vi "SW_Gen_2D_Histogram.vi"(7 "Picture reference in":refnum<vi>, 8 "Pixels per mm":dbl, 9 "Y coord array":dbl[](array[numeric]), 10 "X coord array":dbl[](array[numeric]), 11 "Bounds":T6) -> (1 "8-bit density map":u8[][](array[numeric]), 2 "24-bit pixmap":u32[][](array[numeric]), 3 "Picture":picture)   [LabVIEW 2018, in "Tracker.lvlib"]
uses:
  Tracker.lvlib
  <vilib>/Utility/miscctls.llb/LVBoundsTypeDef.ctl
  <vilib>/Heliosphere Research LLC/Advanced Plotting Toolkit/api_plotting/Histogram2DProperties.ctl
  <vilib>/Heliosphere Research LLC/Advanced Plotting Toolkit/properties/Colormap.ctl
  <vilib>/Heliosphere Research LLC/Advanced Plotting Toolkit/properties/Colormap_Map.ctl
  <vilib>/Heliosphere Research LLC/Advanced Plotting Toolkit/properties/Colormap_Scaling.ctl
  <vilib>/Heliosphere Research LLC/Advanced Plotting Toolkit/properties/Display.ctl
  <vilib>/Heliosphere Research LLC/Advanced Plotting Toolkit/api_plotting/Histogram2DRange.ctl
  <vilib>/Heliosphere Research LLC/Advanced Plotting Toolkit/api_core/NewPlotProperties.ctl
  <vilib>/Heliosphere Research LLC/Advanced Plotting Toolkit/typedefs/PlotColor.ctl
  <vilib>/Heliosphere Research LLC/Advanced Plotting Toolkit/api_core/NewPlotType.ctl
  <vilib>/Heliosphere Research LLC/Advanced Plotting Toolkit/api_plotting/Histogram2D_Automatic.vi
  <vilib>/Heliosphere Research LLC/Advanced Plotting Toolkit/Advanced Plotting Toolkit.lvlib
panel:
  in  "Histogram properties":T1={"Normalize"=TRUE, "Colormap"={"Map"=enum."Rainbow", "Value Min"=nan, "Value Max"=nan, "Scaling"=enum."Default", "Reverse"=FALSE}, "Display"={"Alpha"=1.0, "Z Order"=nan}}
  out "Picture 2":picture
  in  "Histogram 2 properties":T1={"Normalize"=FALSE, "Colormap"={"Map"=enum."Automatic", "Value Min"=nan, "Value Max"=nan, "Scaling"=enum."Default", "Reverse"=FALSE}, "Display"={"Alpha"=nan, "Z Order"=nan}}
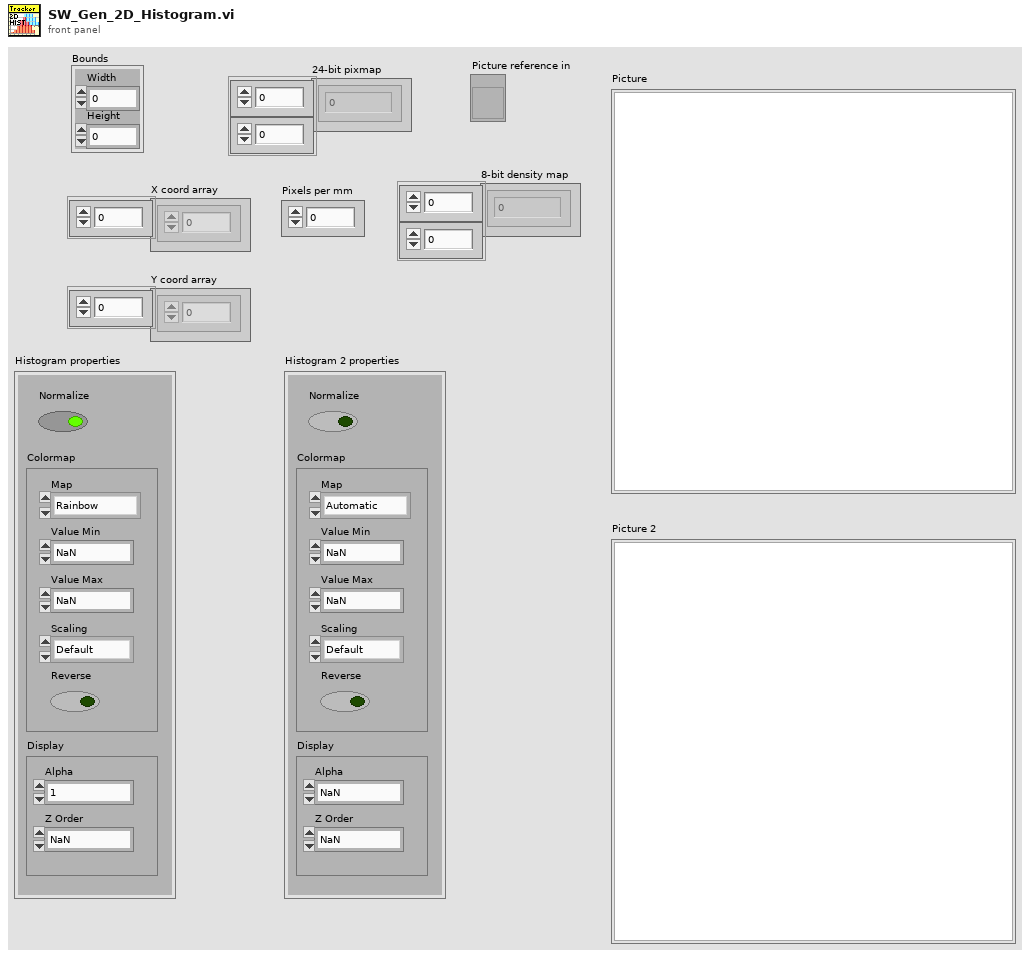
[diagram p1: front panel]
types:
  T1 = typedef "Advanced Plotting Toolkit.lvlib/Histogram2DProperties.ctl" = cluster{"Normalize":bool, "Colormap":T2, "Display":T5}
  T2 = typedef "Advanced Plotting Toolkit.lvlib/Colormap.ctl" = cluster{"Map":T3, "Value Min":dbl, "Value Max":dbl, "Scaling":T4, "Reverse":bool}
  T3 = typedef "Advanced Plotting Toolkit.lvlib/Colormap_Map.ctl" = enum16{"Automatic", "Rainbow", "Hot and Cold", "White-Black", "White-Blue", "White-Green", "White-Red", "Fire", "Water", "Earth", "Air", "Pastel", "Banded", "Stepped"}
  T4 = typedef "Advanced Plotting Toolkit.lvlib/Colormap_Scaling.ctl" = enum16{"Default"}
  T5 = typedef "Advanced Plotting Toolkit.lvlib/Display.ctl" = cluster{"Alpha":dbl, "Z Order":dbl}
  T6 = typedef "LVBoundsTypeDef.ctl" = cluster{"Width":u32, "Height":u32}
  T7 = typedef "Advanced Plotting Toolkit.lvlib/NewPlotType.ctl" = enum16{"Rectangular Axes", "Polar Axes"}
  T8 = typedef "Advanced Plotting Toolkit.lvlib/NewPlotProperties.ctl" = cluster{"Background Color":T9, "Axis Background":T9, "Left Margin":dbl, "Right Margin":dbl, "Bottom Margin":dbl, "Top Margin":dbl, "Aspect Ratio":dbl}
  T9 = typedef "Advanced Plotting Toolkit.lvlib/PlotColor.ctl" = u32
  T10 = typedef "Advanced Plotting Toolkit.lvlib/Histogram2DRange.ctl" = cluster{"X Min":dbl, "X Max":dbl, "Y Min":dbl, "Y Max":dbl}
  T11 = typedef "Advanced Plotting Toolkit.lvlib/PlotID.ctl" = i32
  T12 = typedef "imagedata.ctl" = cluster{"image type":i32, "image depth":i32, "image":u8[], "mask":u8[], "colors":u32[], "Rectangle":cluster{"left":i16, "top":i16, "right":i16, "bottom":i16}}
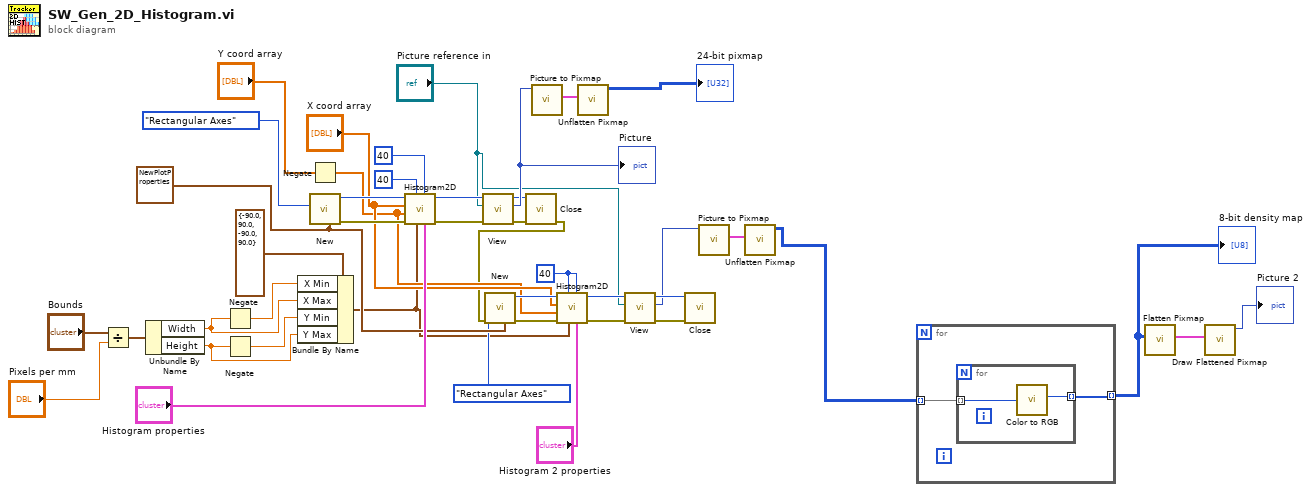
[diagram p0: block diagram]
diagram:
  w15 = 40 ("X Bins")
  w21 = T8 {"Background Color"=2147483647, "Axis Background"=2147483647, "Left Margin"=0.0, "Right Margin"=0.0, "Bottom Margin"=0.0, "Top Margin"=0.0, "Aspect Ratio"=1.0} ("Plot properties")
  n1 = Divide(x="Bounds", y="Pixels per mm") -> (x/y=w39:cluster{"Width":dbl, "Height":dbl})
  n2 = Unbundle By Name(w39) -> ("Width"=w40:dbl, "Height"=w41:dbl)
  n3 = Negate(x=w40) -> (-x=w42:dbl)
  n4 = Negate(x=w41) -> (-x=w43:dbl)
  n5 = Bundle By Name(cluster=T10 {"X Min"=-90.0, "X Max"=90.0, "Y Min"=-90.0, "Y Max"=90.0} ("Data Range"), "X Min"=w42, "X Max"=w40, "Y Min"=w43, "Y Max"=w41) -> (w7:T10)
  n6 = Negate(x="Y coord array") -> (-x=w17:dbl[])
  n7 = call <vilib>:"New.vi"("Properties"=w21, "Plot Type"=NewPlotType."Rectangular Axes") -> ("error out"=w28:errorcluster, "Plot ID"=w26:T11)  [unwired: 8 in]
  n8 = call-poly <vilib>:"Histogram2D.vi"("Properties"="Histogram properties", "Y Bins"=40, "Data Range"=w7, "X Bins"=40, "error in (no error)"=w28, "Y Data"=w17, "X Data"="X coord array", "Plot ID"=w26) -> ("error out"=w29:errorcluster, "Plot ID Out"=w35:T11)  [unwired: 2 in]
  n9 = call <vilib>:"View.vi"("error in (no error)"=w29, "Ref for Sizing"="Picture reference in", "Plot ID"=w35) -> ("error out"=w31:errorcluster, "Picture"=w36:picture, "Plot ID Out"=w30:T11)  [unwired: 6 in]
  "Picture" <- w36
  n10 = call <vilib>:"Close.vi"("error in (no error)"=w31, "Plot ID"=w30) -> ("error out"=w9:errorcluster)  [unwired: 9 in]
  n11 = call <vilib>:"New.vi"("Properties"=w21, "error in (no error)"=w9, "Plot Type"=NewPlotType."Rectangular Axes") -> ("error out"=w8:errorcluster, "Plot ID"=w19:T11)  [unwired: 7 in]
  n12 = call <vilib>:"Picture to Pixmap.vi"("picture"=w36) -> ("image data"=w37:T12)  [unwired: 9 in, 1 out]
  n13 = call-poly <vilib>:"Histogram2D.vi"("Properties"="Histogram 2 properties", "Y Bins"=w15, "Data Range"=w7, "X Bins"=w15, "error in (no error)"=w8, "Y Data"=w17, "X Data"="X coord array", "Plot ID"=w19) -> ("error out"=w14:errorcluster, "Plot ID Out"=w13:T11)  [unwired: 2 in]
  n14 = call <vilib>:"Unflatten Pixmap.vi"("image data"=w37) -> ("24-bit pixmap"=→"24-bit pixmap":u32[][])  [unwired: 4 in, 6 out]
  n15 = call <vilib>:"View.vi"("error in (no error)"=w14, "Ref for Sizing"="Picture reference in", "Plot ID"=w13) -> ("error out"=w12:errorcluster, "Picture"=w3:picture, "Plot ID Out"=w11:T11)  [unwired: 6 in]
  n16 = call <vilib>:"Close.vi"("error in (no error)"=w12, "Plot ID"=w11) -> ()  [unwired: 9 in, 1 out]
  n17 = call <vilib>:"Picture to Pixmap.vi"("picture"=w3) -> ("image data"=w6:T12)  [unwired: 9 in, 1 out]
  n18 = call <vilib>:"Unflatten Pixmap.vi"("image data"=w6) -> ("24-bit pixmap"=w5:u32[][])  [unwired: 4 in, 6 out]
  n19 = for {
    tunnel: w5 -> [w45] mode=indexing
    tunnel: [w44] -> w1 mode=indexing
    n20 = for {
      tunnel: w45 -> [w47] mode=indexing
      tunnel: [w46] -> w44 mode=indexing
      n21 = call <vilib>:"Color to RGB.vi"("Color"=w47) -> ("R"=w46:u8)  [unwired: 3 out]
    }
  }
  "8-bit density map" <- w1
  n22 = call <vilib>:"Flatten Pixmap.vi"("8-bit pixmap"=w1) -> ("image data"=w4:T12)  [unwired: 10 in]
  n23 = call <vilib>:"Draw Flattened Pixmap.vi"("image data"=w4) -> ("new picture"=→"Picture 2":picture)  [unwired: 8 in]
